vi "Update Connection State.vi"(8 "error in (no error)":errorcluster, 10 "Update Connection State Msg":refnum<class "Update Connection State Msg.lvclass">, 11 "CS++GoBangServer in":refnum<class "CS++GoBangServer.lvclass">) -> (0 "error out":errorcluster, 3 "CS++GoBangServer out":refnum<class "CS++GoBangServer.lvclass">)   [LabVIEW 2014, in "GoBang.lvlib" / "CS++GoBangServer.lvclass"]
uses:
  CS++GoBangServer.lvclass
  CS++GoBangServer Messages/Update Connection State Msg/Update Connection State Msg.lvclass
  typdefs/GameState.ctl
  <vilib>/NI/Actors/Linked Network Actor/Linked Network Actor Messages/LNA Connection Status Msg/LNA Connection Status Msg.lvclass/LNA Connection Status Msg.ctl
  CS++GoBangClient Messages/Show Disconnected Msg Msg/Show Disconnected Msg Msg.lvclass
  CS++GoBangServer.lvclass/CS++GoBangServer.ctl
  <vilib>/NI/Actors/Linked Network Actor/Linked Network Actor Messages/LNA Connection Status Msg/LNA Connection Status Msg.lvclass
  GoBang.lvlib
  <vilib>/NI/Actors/Linked Network Actor/Linked Network Actor Messages/Transmit Network Message Msg/Transmit Network Message Msg.lvclass
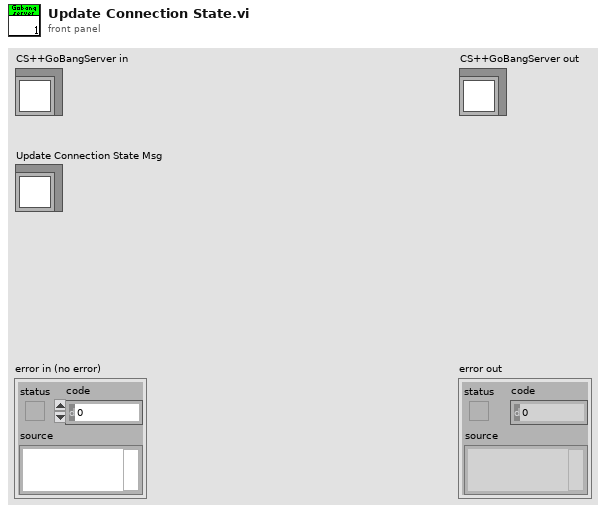
[diagram p1: front panel]
types:
  T1 = typedef "GoBang.lvlib/GameState.ctl" = enum16{"Waiting for opponent", "White to move", "Black to move", "Game over, white won", "Game over, black won"}
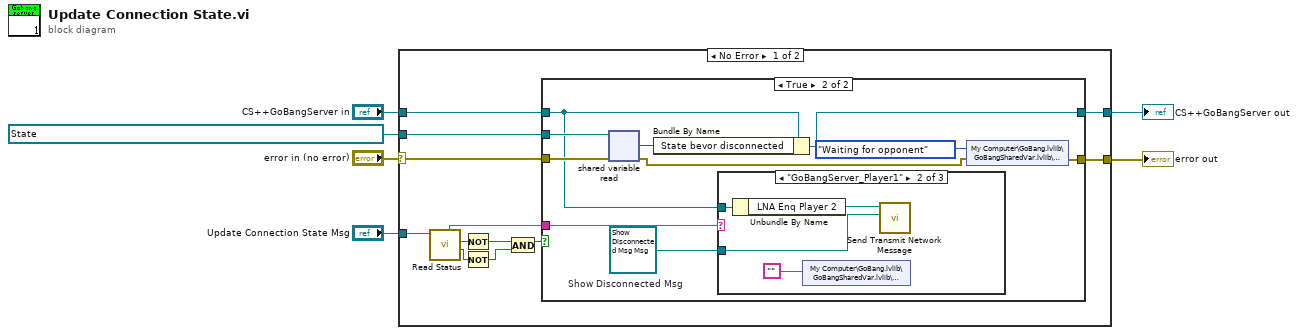
[diagram p0: block diagram]
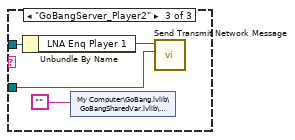
[diagram p4: hidden frame]
diagram:
  w1 = refnum<k21> "ni.var.psp://My Computer/GoBang/GoBangSharedVar/GameState" items=["Waiting for opponent", "White to move", "Black to move", "Game over, white won", "Game over, black won"] ("shared variable refnum in")
  n1 = case shown="No Error" "error in (no error)" {
    selector: "error in (no error)" -> [w12 w40]
    tunnel: [w11 w40] -> w5
    tunnel: [w13 w39] -> w3
    tunnel: "CS++GoBangServer in" -> [w14 w39]
    tunnel: "Update Connection State Msg" -> [w18 _]
    tunnel: w1 -> [w15 _]
    frame No Error {
      n2 = call <vilib>:"Read Status.vi"("Update Status Msg in"=w18) -> ("Reader"=w9:bool, "Writer"=w16:bool, "Name"=w17:string)  [unwired: 7 in, 1 out]
      n3 = Not(x=w16) -> (.not. x?=w10:bool)
      n4 = Not(x=w9) -> (.not. x?=w7:bool)
      n5 = And(x=w10, y=w7) -> (x .and. y?=w8:bool)
      n6 = case shown="True" w8 {
        tunnel: w17 -> [_ w29]
        tunnel: w15 -> [_ w28]
        tunnel: w14 -> [w20 w22]
        tunnel: [w20 w26] -> w13
        tunnel: w12 -> [w19 w24]
        tunnel: [w19 w23] -> w11
        frame False {
        }
        frame True {
          w21 = refnum<class "Show Disconnected Msg Msg.lvclass"> refnum  # Show Disconnected Msg
          n7 = shared-variable-read(w28, w24) -> (w25:errorcluster, w27:T1)  [unwired: 1 out]
          n8 = Bundle By Name(cluster=w22, "State bevor disconnected"=w27) -> (w26:refnum<class "CS++GoBangServer.lvclass">)
          n9 = case shown="\"GoBangServer_Player1\"" w29 {
            tunnel: w22 -> [_ w32 w37]
            tunnel: w21 -> [_ w31 w35]
            frame "False", Default {
            }
            frame "GoBangServer_Player1" {
              n10 = Unbundle By Name(w32) -> ("LNA Enq Player 2"=w33:refnum<class "Message Enqueuer.lvclass">)
              n11 = shared-variable "My Computer\\GoBang.lvlib\\GoBangSharedVar.lvlib\\WhitePlayer"("") -> ()  [unwired: 1 in, 1 out]
              n12 = call <vilib>:"Send Transmit Network Message.vi"("Message"=w31, "Message Enqueuer"=w33) -> ()  [unwired: 8 in, 2 out]
            }
            frame "GoBangServer_Player2" {
              n13 = Unbundle By Name(w37) -> ("LNA Enq Player 1"=w36:refnum<class "Message Enqueuer.lvclass">)
              n14 = shared-variable "My Computer\\GoBang.lvlib\\GoBangSharedVar.lvlib\\BlackPlayer"("") -> ()  [unwired: 1 in, 1 out]
              n15 = call <vilib>:"Send Transmit Network Message.vi"("Message"=w35, "Message Enqueuer"=w36) -> ()  [unwired: 8 in, 2 out]
            }
          }
          n16 = shared-variable "My Computer\\GoBang.lvlib\\GoBangSharedVar.lvlib\\GameState"(GameState."Waiting for opponent" ("GameState"), error in=w25) -> (error out=w23:errorcluster)
        }
      }
    }
    frame Error {
    }
  }
  "error out" <- w5
  "CS++GoBangServer out" <- w3
